vi "Host.vi"() -> ()   [LabVIEW 2019]
panel:
  out "Waveform Chart":i32(graph)
  in  "HF:Enable E-Stop":bool
  in  "HG:Drive Direction":i16
  out "FH:DriveFa":bool
  out "FH:DriveStatus":i32
  out "GH:Current Sense":i32
  in  "HF:Motor":bool=TRUE
  out "FH:Vsup Present":bool
  in  "stop":bool
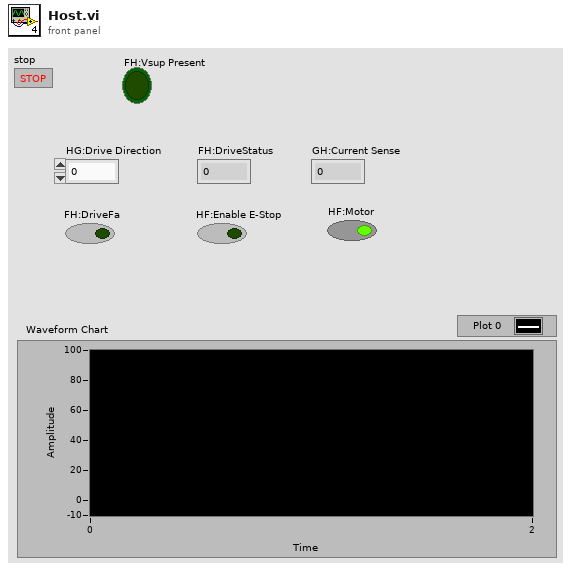
[diagram p1: front panel]
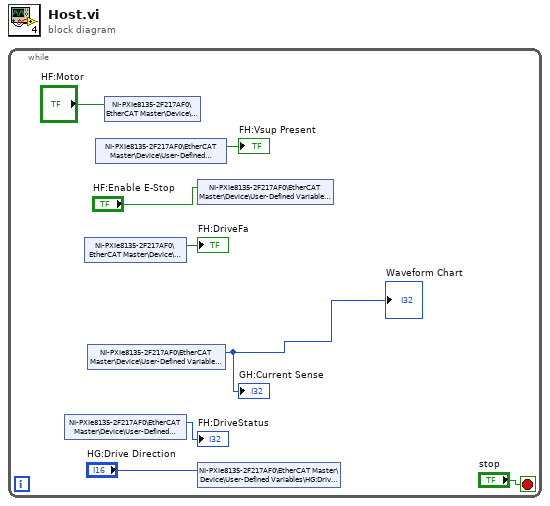
[diagram p0: block diagram]
diagram:
  n1 = while {
    stop <- "stop" stop-if-true
    n2 = shared-variable "NI-PXIe8135-2F217AF0\\EtherCAT Master\\Device\\User-Defined Variables\\FH:DriveStatus"() -> (→"FH:DriveStatus":i32)  [unwired: 1 in, 1 out]
    n3 = shared-variable "NI-PXIe8135-2F217AF0\\EtherCAT Master\\Device\\User-Defined Variables\\FH:DriveFa"() -> (→"FH:DriveFa":bool)  [unwired: 1 in, 1 out]
    n4 = shared-variable "NI-PXIe8135-2F217AF0\\EtherCAT Master\\Device\\User-Defined Variables\\GH:Current Sense"() -> (→"GH:Current Sense" →"Waveform Chart":i32)  [unwired: 1 in, 1 out]
    n5 = shared-variable "NI-PXIe8135-2F217AF0\\EtherCAT Master\\Device\\User-Defined Variables\\FH:Vsup Present"() -> (→"FH:Vsup Present":bool)  [unwired: 1 in, 1 out]
    n6 = shared-variable "NI-PXIe8135-2F217AF0\\EtherCAT Master\\Device\\User-Defined Variables\\HF:Motor"("HF:Motor") -> ()  [unwired: 1 in, 1 out]
    n7 = shared-variable "NI-PXIe8135-2F217AF0\\EtherCAT Master\\Device\\User-Defined Variables\\HF:Enable E-Stop"("HF:Enable E-Stop") -> ()  [unwired: 1 in, 1 out]
    n8 = shared-variable "NI-PXIe8135-2F217AF0\\EtherCAT Master\\Device\\User-Defined Variables\\HG:Drive Direction"("HG:Drive Direction") -> ()  [unwired: 1 in, 1 out]
  }
